vi "TubingCompensation.vi"(7 "NyquistLimitedCoefficients":dbl[](array[numeric]), 9 "NyquistLimitedPhase":dbl[](array[numeric]), 10 "mutedData":dbl[](array[numeric]), 11 "SamplingFreq":dbl) -> (2 "boostedData":dbl[](array[numeric]))   [LabVIEW 2012]
uses:
  <vilib>/Analysis/NI_AALBase.lvlib
panel:
  out "SDincrease(%)":dbl format="%.1f"
  out "Waveform Graph":dbl[][](graph)
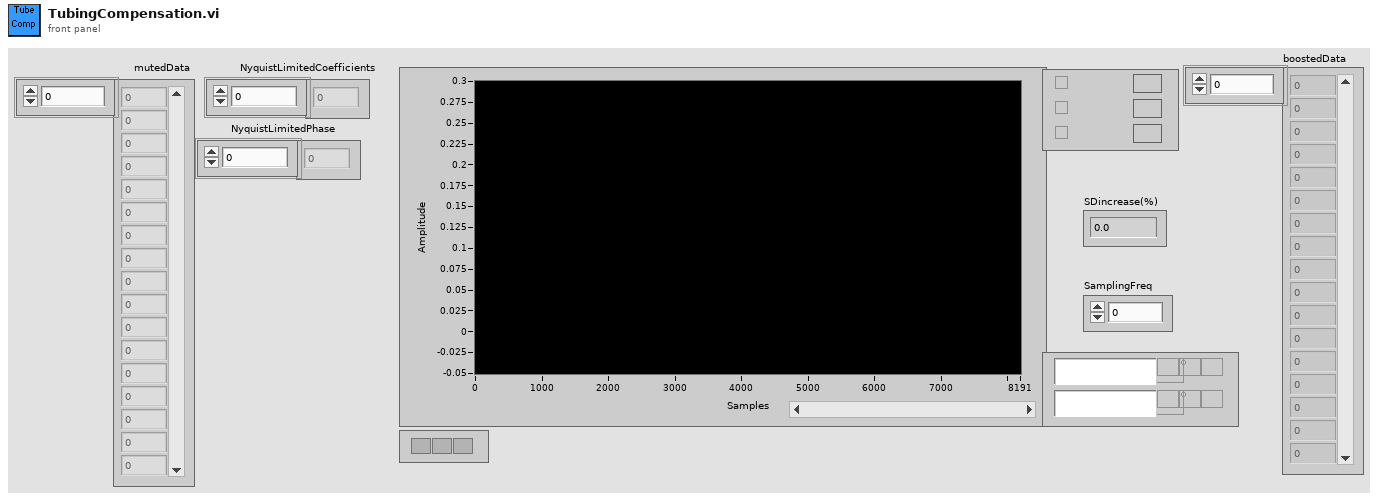
[diagram p1: front panel]
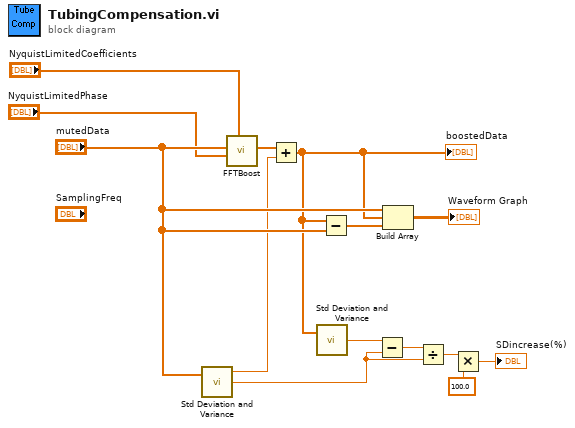
[diagram p0: block diagram]
diagram:
  n1 = call <vilib>:"Std Deviation and Variance.vi"("X"="mutedData") -> ("mean"=w3:dbl, "standard deviation"=w8:dbl)  [unwired: 1 in, 1 out]
  n2 = call "FFTBoost.vi"("CompensationCoefficients"="NyquistLimitedCoefficients", "PhaseCorrection"="NyquistLimitedPhase", "mutedData"="mutedData") -> ("boostedData"=w11:dbl[])  [unwired: 1 in, 7 out]
  n3 = Add(x=w11, y=w3) -> (x+y=w4:dbl[])
  "boostedData" <- w4
  n4 = call <vilib>:"Std Deviation and Variance.vi"("X"=w4) -> ("standard deviation"=w10:dbl)  [unwired: 1 in, 2 out]
  n5 = Subtract(x=w4, y="mutedData") -> (x-y=w13:dbl[])
  n6 = Subtract(x=w10, y=w8) -> (x-y=w9:dbl)
  n7 = Build Array("mutedData", w4, w13) -> (→"Waveform Graph":dbl[][])
  n8 = Divide(x=w9, y=w8) -> (x/y=w7:dbl)
  n9 = Multiply(x=w7, y=100.0) -> (x*y=→"SDincrease(%)":dbl)
